vi "Autonomous Independent.vi"() -> ()   [LabVIEW 2013]
doc: "This VI is called when autonomous begins, and will automatically be terminated when autonomous ends. You can carry out timed or sensor driven robot movement independently without needing to return to the caller."
uses:
  <vilib>/Rock Robotics/WPI/DriverStation/WPI_DriverStationMatch Info.ctl
  <vilib>/Rock Robotics/WPI/Solenoid/WPI_SolenoidValue.ctl
  <vilib>/Rock Robotics/WPI/Relay/WPI_RelayValue.ctl
  Robot Global Data.vi
  <vilib>/Rock Robotics/WPI/RobotDrive/WPI_RobotDriveArcadeDrive_Standard(NoSaturation).vi
  <vilib>/Rock Robotics/WPI/RobotDrive/WPI_RobotDriveGetSetRefNum.vi
  <vilib>/Rock Robotics/WPI/Solenoid/WPI_SolenoidSetEnum.vi
panel:
  in  "Match Info":T1={"Autonomous Elapsed Seconds"=0.0, "TeleOp Elapsed Seconds"=0.0, "Disabled Elapsed Seconds"=0.0, "Visited Autonomous"=FALSE, "Visited TeleOp"=FALSE, "Visited Disabled"=FALSE, "Autonomous Settings"={"Autonomous Style"=enum."Independent", "VI Refnum"=refnum}}
  # "Be sure to right-click and choose Data Operations>>Make Current Value default if you want to save the array values with the VI"
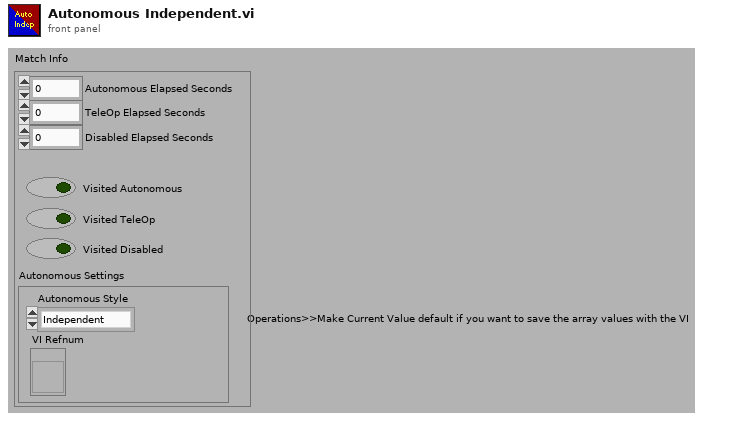
[diagram p1: front panel]
types:
  T1 = typedef "WPI_DriverStationMatch Info.ctl" = cluster{"Autonomous Elapsed Seconds":dbl, "TeleOp Elapsed Seconds":dbl, "Disabled Elapsed Seconds":dbl, "Visited Autonomous":bool, "Visited TeleOp":bool, "Visited Disabled":bool, "Autonomous Settings":cluster{"Autonomous Style":enum16{"Iterative", "Independent"}, "VI Refnum":refnum<vi>}}
  T2 = typedef "WPI_SolenoidValue.ctl" = enum16{"Off", "On", "Forward", "Reverse"}
  T3 = typedef "WPI_RelayValue.ctl" = enum16{"Off", "On", "Forward", "Reverse"}
  T4 = typedef "WPI_RobotDriveDevRef.ctl" = cluster{"DevStatus":errorcluster, "Motors[]":T5[], "Square Inputs":bool, "Max Output":dbl, "Isochronous":bool}
  T5 = typedef "WPI_MotorControlDeviceRef.ctl" = cluster{"DeviceStatus":errorcluster, "Type":enum16{"PWM", "CAN"}, "PWM":cluster{"Digital Module":T6, "PWM Channel":T7, "DeadBand":T8}, "CAN":cluster{"Device Number":u8, "Control Mode":T9, "Semaphore":T10, "Max Vout":dbl}, "Invert":bool, "TransformRef":T11, "InvTransformRef":T11}
  T6 = typedef "FPGA_TypedefDigitalModule.ctl" = enum16{"Digital Module 1", "Digital Module 2"}
  T7 = typedef "FPGA_DIOPWMChannel.ctl" = enum8{"PWM 1", "PWM 2", "PWM 3", "PWM 4", "PWM 5", "PWM 6", "PWM 7", "PWM 8", "PWM 9", "PWM 10", "Invalid"}
  T8 = typedef "WPI_PWMDeadband.ctl" = cluster{"Name":string, "maxPositivePwm":i32, "minPositivePwm":i32, "centerPwm":i32, "maxNegativePwm":i32, "minNegativePwm":i32, "angularRange":u16}
  T9 = typedef "WPI_CANJaguar_ControlMode.ctl" = enum8{"Percent VBus", "Current", "Speed", "Position", "Voltage"}
  T10 = typedef "Semaphore RefNum" = refnum<k1>
  T11 = typedef "WPI_PWMTransform_ConPane.ctl" = refnum<vi>
  T12 = typedef "WPI_SolenoidDevRef.ctl" = cluster{"DevStatus":errorcluster, "Solenoid Module":T13, "Forward Solenoid Channel":T14, "Reverse Solenoid Channel":T14}
  T13 = typedef "FPGA_TypedefSolenoidModule.ctl" = enum16{"Solenoid Module 1", "Solenoid Module 2"}
  T14 = typedef "WPI_SolenoidChannel.ctl" = enum8{"Solenoid 1", "Solenoid 2", "Solenoid 3", "Solenoid 4", "Solenoid 5", "Solenoid 6", "Solenoid 7", "Solenoid 8", "Invalid"}
  T15 = typedef "WPI_RelayDevRef.ctl" = cluster{"DevStatus":errorcluster, "Relay Channel":T16, "Digital Module":T6, "Relay Direction":T17}
  T16 = typedef "FPGA_DIORelayChannel.ctl" = enum8{"Relay 1", "Relay 2", "Relay 3", "Relay 4", "Relay 5", "Relay 6", "Relay 7", "Relay 8", "Invalid"}
  T17 = typedef "WPI_RelayDirection.ctl" = enum16{"Both directions", "Forward only", "Reverse only"}
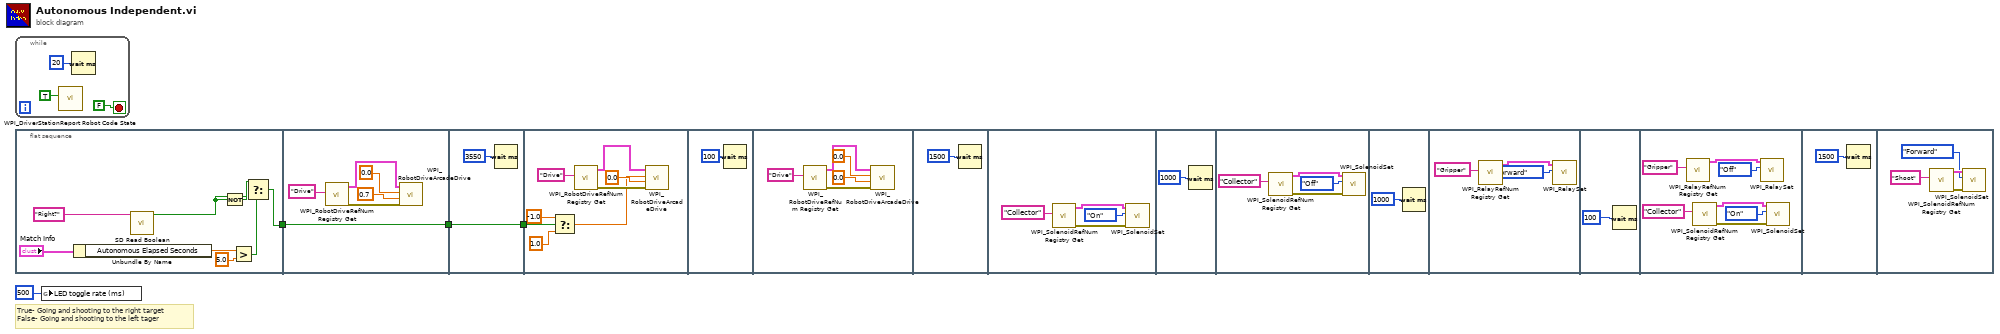
[diagram p0: block diagram]
diagram:
  # "True- Going and shooting to the right target\nFalse- Going and shooting to the left tager"
  n1 = while {
    stop <- FALSE stop-if-true
    n2 = call <vilib>:"WPI_DriverStationReport Robot Code State.vi"("Autonomous"=TRUE) -> ()  [unwired: 10 in, 1 out]
    n3 = Wait (ms)(milliseconds to wait=u32 20) -> ()  [unwired: 1 out]
  }
  n4 = flat-sequence {
    tunnel: [w8] -> w1
    tunnel: [w16] -> w2
    tunnel: w1 -> [w16]
    tunnel: [w22] -> w3
    tunnel: w2 -> [w22]
    tunnel: w3 -> [w27]
    frame #0 {
      n5 = Unbundle By Name("Match Info") -> ("Autonomous Elapsed Seconds"=w10:dbl)
      n6 = call <vilib>:"SD Read Boolean.vi"("Name"="Right?") -> ("Boolean"=w14:bool)  [unwired: 8 in, 2 out]
      n7 = Not(x=w14) -> (.not. x?=w15:bool)
      n8 = Greater?(x=w10, y=5.0) -> (0:w13:bool)
      n9 = Select(t=w15, s=w13, f=w14) -> (s? t:f=w8:bool)
    }
    frame #1 {
      n10 = call <vilib>:"WPI_RobotDriveRefNum Registry Get.vi"("refnum name"="Drive") -> ("error out"=w18:errorcluster, "RobotDriveDevRef"=w17:T4)  [unwired: 9 in]
      n11 = call-poly <vilib>:"WPI_RobotDriveArcadeDrive.vi"("error in (no error)"=w18, "Y axis value"=0.7, "X axis value"=0.0, "RobotDriveDevRef"=w17) -> ()  [unwired: 3 in, 5 out]
    }
    frame #2 {
      n12 = Wait (ms)(milliseconds to wait=3550) -> ()  [unwired: 1 out]
    }
    frame #3 {
      n13 = Select(t=-1.0, s=w27, f=1.0 ("t")) -> (s? t:f=w24:dbl)
      n14 = call <vilib>:"WPI_RobotDriveRefNum Registry Get.vi"("refnum name"="Drive") -> ("error out"=w30:errorcluster, "RobotDriveDevRef"=w31:T4)  [unwired: 9 in]
      n15 = call-poly <vilib>:"WPI_RobotDriveArcadeDrive.vi"("error in (no error)"=w30, "Y axis value"=0.0, "X axis value"=w24, "RobotDriveDevRef"=w31) -> ()  [unwired: 3 in, 5 out]
    }
    frame #4 {
      n16 = Wait (ms)(milliseconds to wait=100) -> ()  [unwired: 1 out]
    }
    frame #5 {
      n17 = call <vilib>:"WPI_RobotDriveRefNum Registry Get.vi"("refnum name"="Drive") -> ("error out"=w34:errorcluster, "RobotDriveDevRef"=w33:T4)  [unwired: 9 in]
      n18 = call-poly <vilib>:"WPI_RobotDriveArcadeDrive.vi"("error in (no error)"=w34, "Y axis value"=0.0, "X axis value"=0.0, "RobotDriveDevRef"=w33) -> ()  [unwired: 3 in, 5 out]
    }
    frame #6 {
      n19 = Wait (ms)(milliseconds to wait=1500) -> ()  [unwired: 1 out]
    }
    frame #7 {
      n20 = call <vilib>:"WPI_SolenoidRefNum Registry Get.vi"("refnum name"="Collector") -> ("error out"=w41:errorcluster, "SolenoidDevRef"=w42:T12)  [unwired: 9 in]
      n21 = call-poly <vilib>:"WPI_SolenoidSet.vi"("error in (no error)"=w41, "Value"=WPI_SolenoidValue."On", "SolenoidDevRef"=w42) -> ()  [unwired: 7 in, 2 out]
    }
    frame #8 {
      n22 = Wait (ms)(milliseconds to wait=1000) -> ()  [unwired: 1 out]
    }
    frame #9 {
      n23 = call <vilib>:"WPI_SolenoidRefNum Registry Get.vi"("refnum name"="Collector") -> ("error out"=w45:errorcluster, "SolenoidDevRef"=w44:T12)  [unwired: 9 in]
      n24 = call-poly <vilib>:"WPI_SolenoidSet.vi"("error in (no error)"=w45, "Value"=WPI_SolenoidValue."Off", "SolenoidDevRef"=w44) -> ()  [unwired: 7 in, 2 out]
    }
    frame #10 {
      n25 = Wait (ms)(milliseconds to wait=1000) -> ()  [unwired: 1 out]
    }
    frame #11 {
      n26 = call <vilib>:"WPI_RelayRefNum Registry Get.vi"("refnum name"="Gripper") -> ("RelayDevRef"=w51:T15)  [unwired: 9 in, 1 out]
      n27 = call <vilib>:"WPI_RelaySet.vi"("RelayValue"=WPI_RelayValue."Forward", "RelayDevRef"=w51) -> ()  [unwired: 8 in, 2 out]
    }
    frame #12 {
      n28 = Wait (ms)(milliseconds to wait=100) -> ()  [unwired: 1 out]
    }
    frame #13 {
      n29 = call <vilib>:"WPI_RelayRefNum Registry Get.vi"("refnum name"="Gripper") -> ("RelayDevRef"=w53:T15)  [unwired: 9 in, 1 out]
      n30 = call <vilib>:"WPI_SolenoidRefNum Registry Get.vi"("refnum name"="Collector") -> ("error out"=w58:errorcluster, "SolenoidDevRef"=w59:T12)  [unwired: 9 in]
      n31 = call <vilib>:"WPI_RelaySet.vi"("RelayValue"=WPI_RelayValue."Off", "RelayDevRef"=w53) -> ()  [unwired: 8 in, 2 out]
      n32 = call-poly <vilib>:"WPI_SolenoidSet.vi"("error in (no error)"=w58, "Value"=WPI_SolenoidValue."On", "SolenoidDevRef"=w59) -> ()  [unwired: 7 in, 2 out]
    }
    frame #14 {
      n33 = Wait (ms)(milliseconds to wait=1500) -> ()  [unwired: 1 out]
    }
    frame #15 {
      n34 = call <vilib>:"WPI_SolenoidRefNum Registry Get.vi"("refnum name"="Shoot") -> ("error out"=w63:errorcluster, "SolenoidDevRef"=w62:T12)  [unwired: 9 in]
      n35 = call-poly <vilib>:"WPI_SolenoidSet.vi"("error in (no error)"=w63, "Value"=WPI_SolenoidValue."Forward", "SolenoidDevRef"=w62) -> ()  [unwired: 7 in, 2 out]
    }
  }
  n36 = global write "Robot Global Data.vi" "LED toggle rate (ms)"(u32 500 ("LED ms toggle rate")) -> ()
